vi "Log status.vi"(8 "entrée d'erreur":errorcluster, 9 "Event Data String (-)":string, 10 "Event string":string, 11 "Log File Refnum In":refnum<file>) -> (0 "error out":errorcluster, 3 "Log File Refnum out":refnum<file>)   [LabVIEW 2017, in "Logging.lvlib"]
doc: "Ce VI enregistre dans un fichier les évènements liés à un appareil. exemple : allumage de l'appareil\nIl enregistre la date et l'heure de l'évènement, sa dénomination et les données qui lui sont liés.\nexemple \n12/12/12 16:45 laser Apmplifier activé"
uses:
  Logging.lvlib
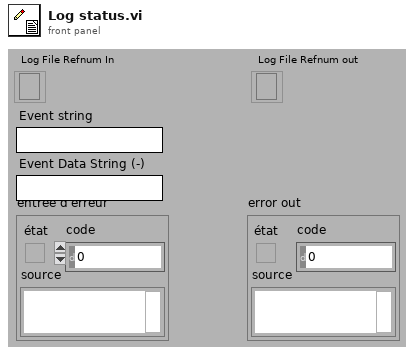
[diagram p1: front panel]
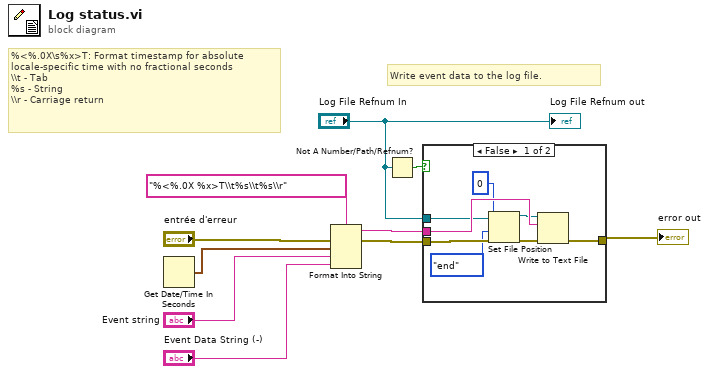
[diagram p0: block diagram]
diagram:
  # "%<%.0X\\s%x>T: Format timestamp for absolute locale-specific time with no fractional seconds\n\\\\t - Tab\n%s - String\n\\\\r - Carriage return"
  # "Write event data to the log file."
  n1 = Get Date/Time In Seconds() -> (seconds since 1Jan1904=w6:timestamp)
  n2 = Format Into String(format string="%<%.0X %x>T\\t%s\\t%s\\r" ("chaîne de format"), error in="entrée d'erreur", w6, "Event string", "Event Data String (-)") -> (resulting string=w3:string, error out=w7:errorcluster)  [unwired: 1 in]
  n3 = Not A Number/Path/Refnum?(number/path/refnum="Log File Refnum In") -> (NaN/Path/Refnum?=w10:bool)
  n4 = case shown="False" w10 {
    tunnel: "Log File Refnum In" -> [w12 _]
    tunnel: w7 -> [w17 w18]
    tunnel: w3 -> [w16 _]
    tunnel: [w15 w18] -> w2
    frame False {
      n5 = Set File Position(offset (in bytes) (0)=i64 0 ("offset (en octets) (0)"), refnum=w12, from (0:start)=enum16{"start", "end", "current"}."end" ("à partir de (0 : start)")) -> (refnum out=w11:refnum<file>)  [unwired: 1 in, 1 out]
      n6 = Write to Text File(file (use dialog)=w11, text=w16, error in=w17) -> (error out=w15:errorcluster)  [unwired: 1 in, 2 out]
    }
    frame True {
    }
  }
  "error out" <- w2
  "Log File Refnum out" <- "Log File Refnum In"
